vi "speech.vi"() -> ()   [LabVIEW 2012]
uses:
  <vilib>/express/express analysis/Spectral/Block/exnSpectralBlock spectral measurements peak poly.vi
  <vilib>/express/express analysis/Spectral/Block/exnSpectralBlock spectral measurements peak DDT.vi
  <vilib>/express/express analysis/Spectral/XNode/ExpressSpectralMeasurementsBlockNode.xnode
panel:
  out "Waveform Graph":dynamicdata(graph)
  in  "Sample rate (Hz)":dbl=20563.01020408163
  in  "Duration (s)":dbl=1.0
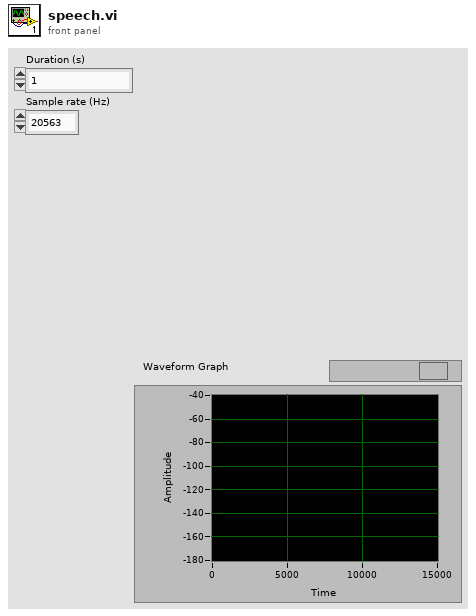
[diagram p1: front panel]
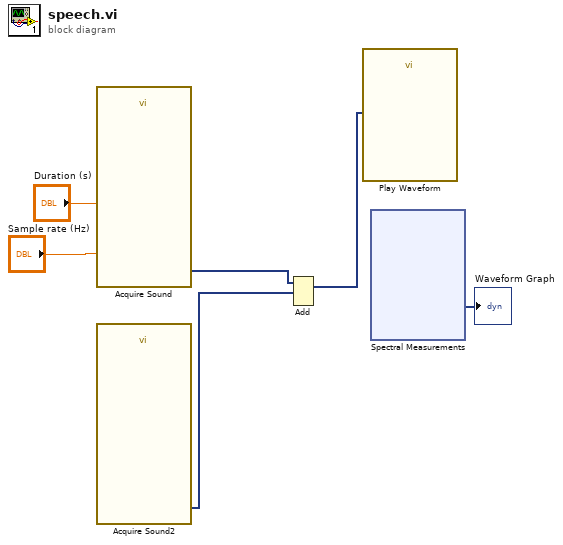
[diagram p0: block diagram]
diagram:
  n1 = call "Acquire Sound"("Duration (s)"="Duration (s)", "Sample rate (Hz)"="Sample rate (Hz)") -> ("Data"=w3:dynamicdata)  [unwired: 16 in, 1 out]
  n2 = call "Acquire Sound2"() -> ("Data"=w2:dynamicdata)  [unwired: 18 in, 1 out]
  n3 = Add(1:w2, 2:w3) -> (0:w1:dynamicdata)  [unwired: 1 in, 1 out]
  n4 = call "Play Waveform"("Data"=w1) -> ()  [unwired: 18 in, 1 out]
  n5 = xnode "Spectral Measurements"() -> ("FFT - (Peak)"=→"Waveform Graph":dynamicdata)  [unwired: 2 in, 2 out]
